vi "AB_900_1000_Project_App_Info.vi"(6 "dataForPrevious in":T1, 7 "action":T2, 8 "error in (no error)":errorcluster, 10 "applicationInfo in":T3, 11 "Object In":T4) -> (0 "error out":errorcluster, 2 "Application info":T3, 3 "Object Out":T4, 4 "dataFromPrevious":T1)   [LabVIEW 2020]
uses:
  <resource>/Framework/Providers/API/ItemRef.ctl
  <vilib>/AppBuilder/RW_Project/AB_RW_Project_PropBag_Action.ctl
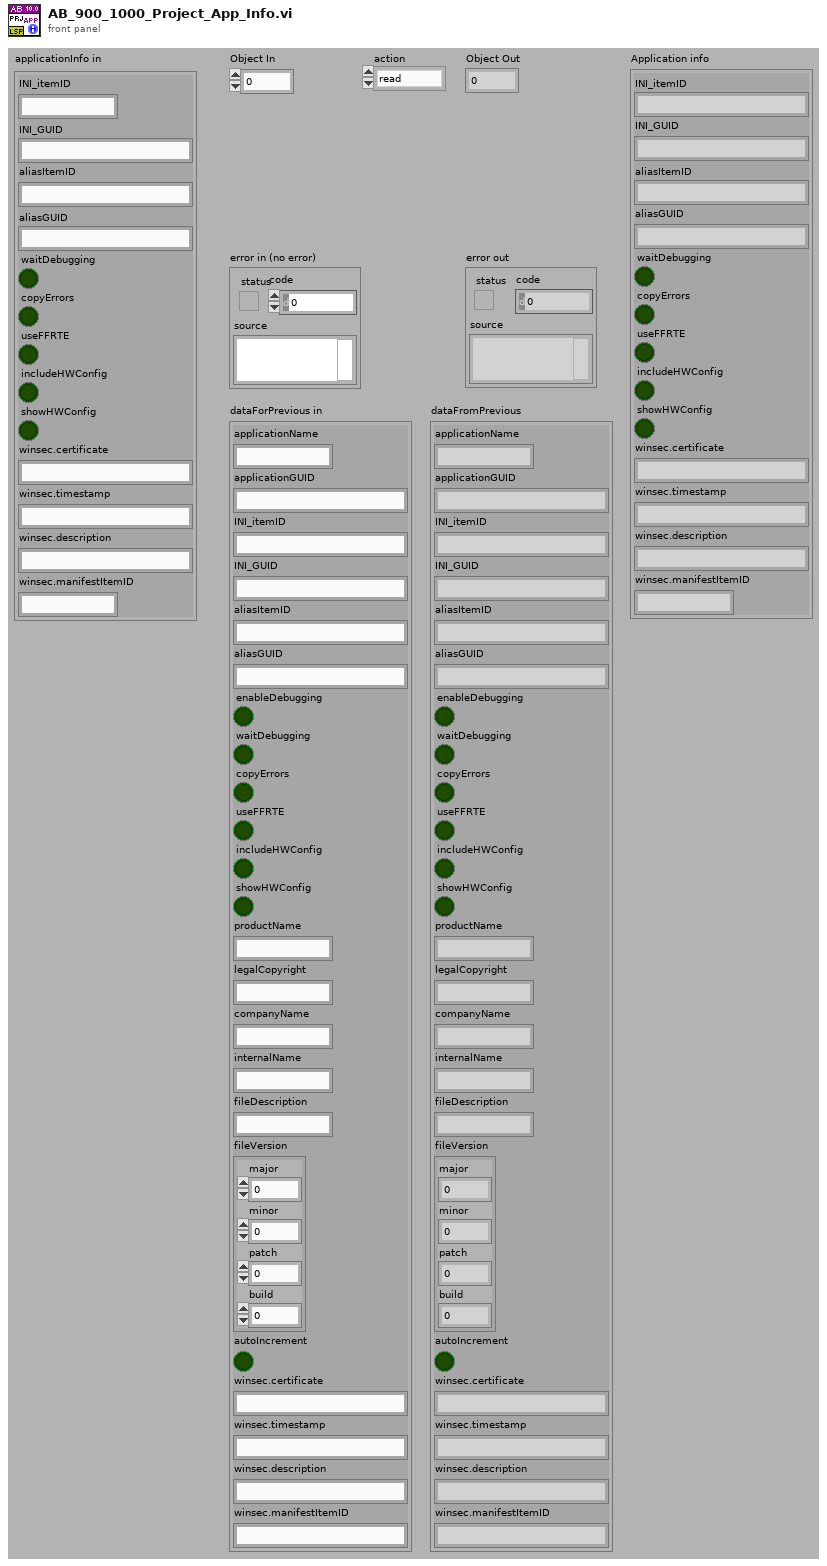
[diagram p1: front panel]
types:
  T1 = cluster{"applicationName":string, "applicationGUID":string, "INI_itemID":string, "INI_GUID":string, "aliasItemID":string, "aliasGUID":string, "enableDebugging":bool, "waitDebugging":bool, "copyErrors":bool, "useFFRTE":bool, "includeHWConfig":bool, "showHWConfig":bool, "productName":string, "legalCopyright":string, "companyName":string, "internalName":string, "fileDescription":string, "fileVersion":cluster{"major":u16, "minor":u16, "patch":u16, "build":u16}, "autoIncrement":bool, "winsec.certificate":string, "winsec.timestamp":string, "winsec.description":string, "winsec.manifestItemID":string}
  T2 = typedef "AB_RW_Project_PropBag_Action.ctl" = enum16{"read", "write", "clear", "readPrevious", "writePrevious", "clearPrevious"}
  T3 = cluster{"INI_itemID":string, "INI_GUID":string, "aliasItemID":string, "aliasGUID":string, "waitDebugging":bool, "copyErrors":bool, "useFFRTE":bool, "includeHWConfig":bool, "showHWConfig":bool, "winsec.certificate":string, "winsec.timestamp":string, "winsec.description":string, "winsec.manifestItemID":string}
  T4 = typedef "ItemRef.ctl" = u64
  T5 = cluster{"[0]":i32, "[1]":i32, "[2]":i32, "[3]":i32}
  T6 = cluster{"major":u16, "minor":u16, "patch":u16, "build":u16}
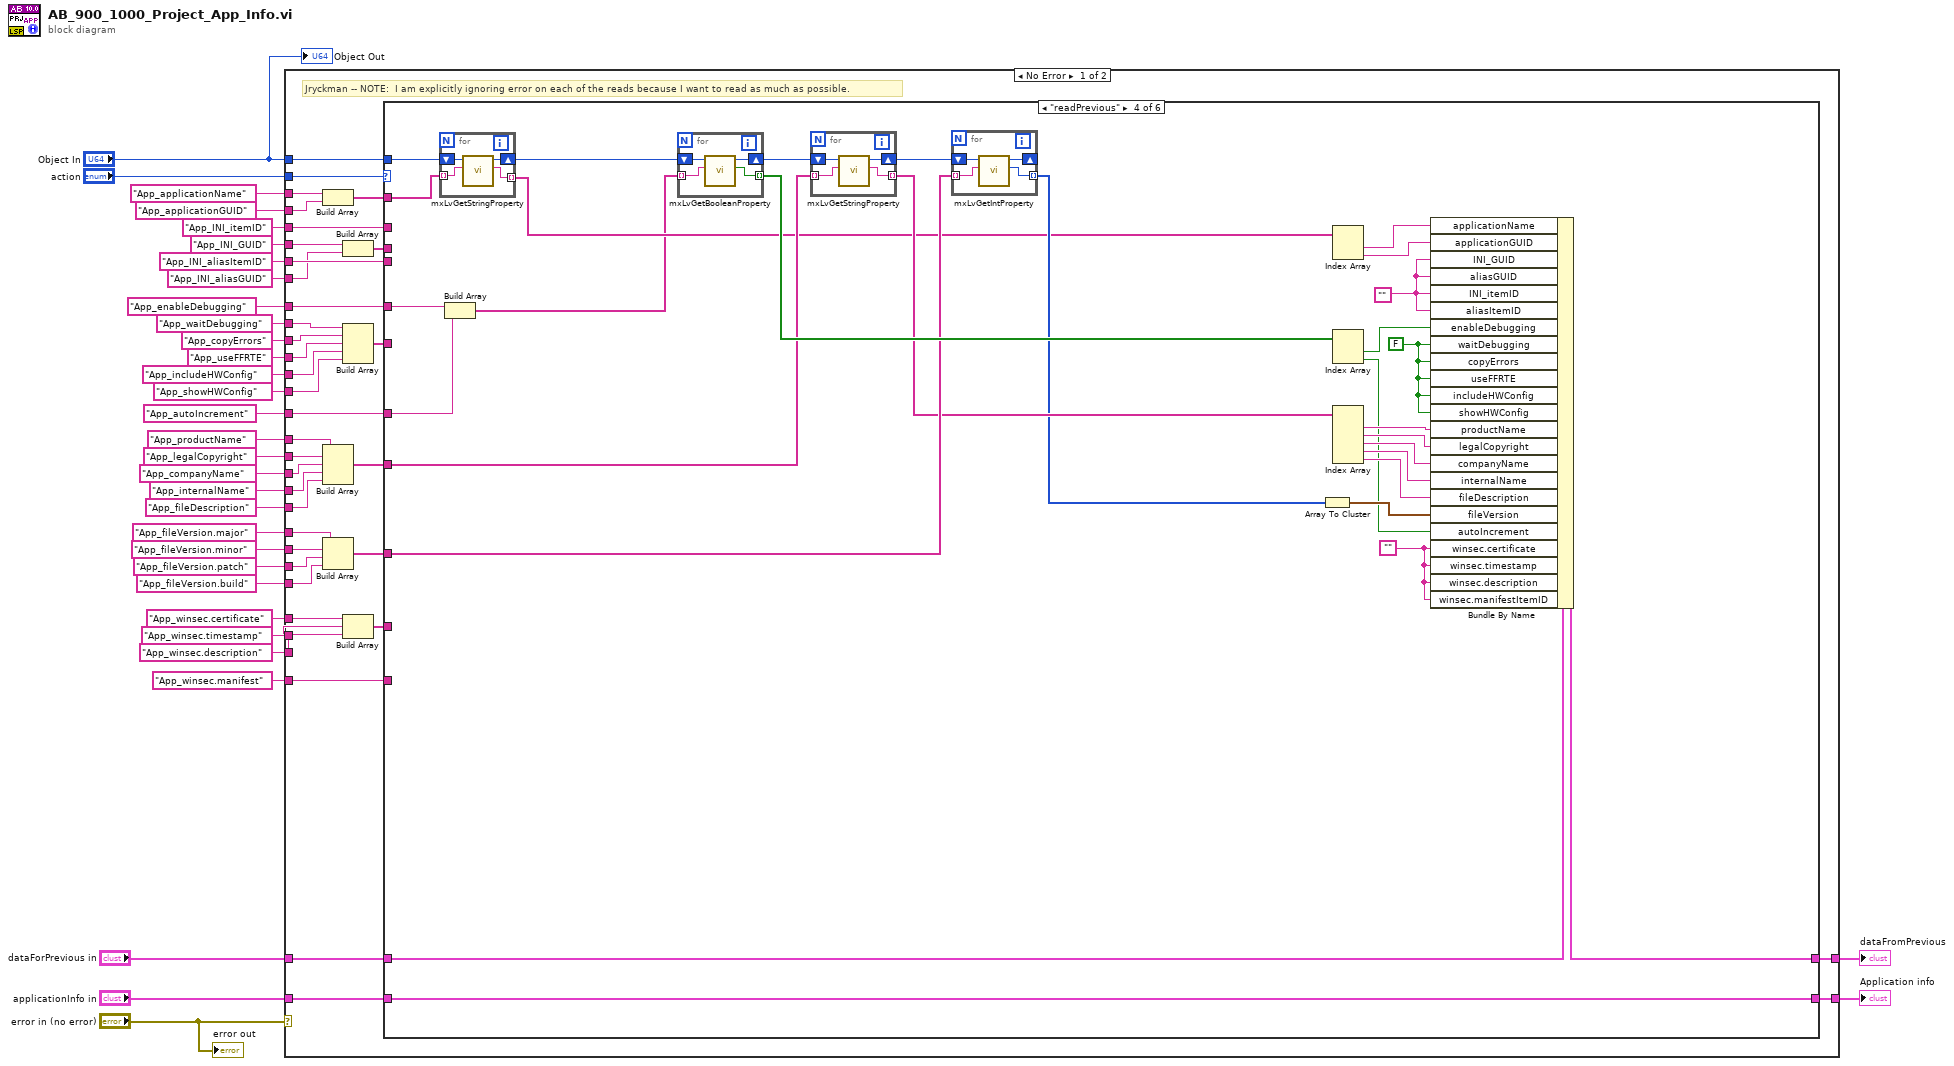
[diagram p0: block diagram]
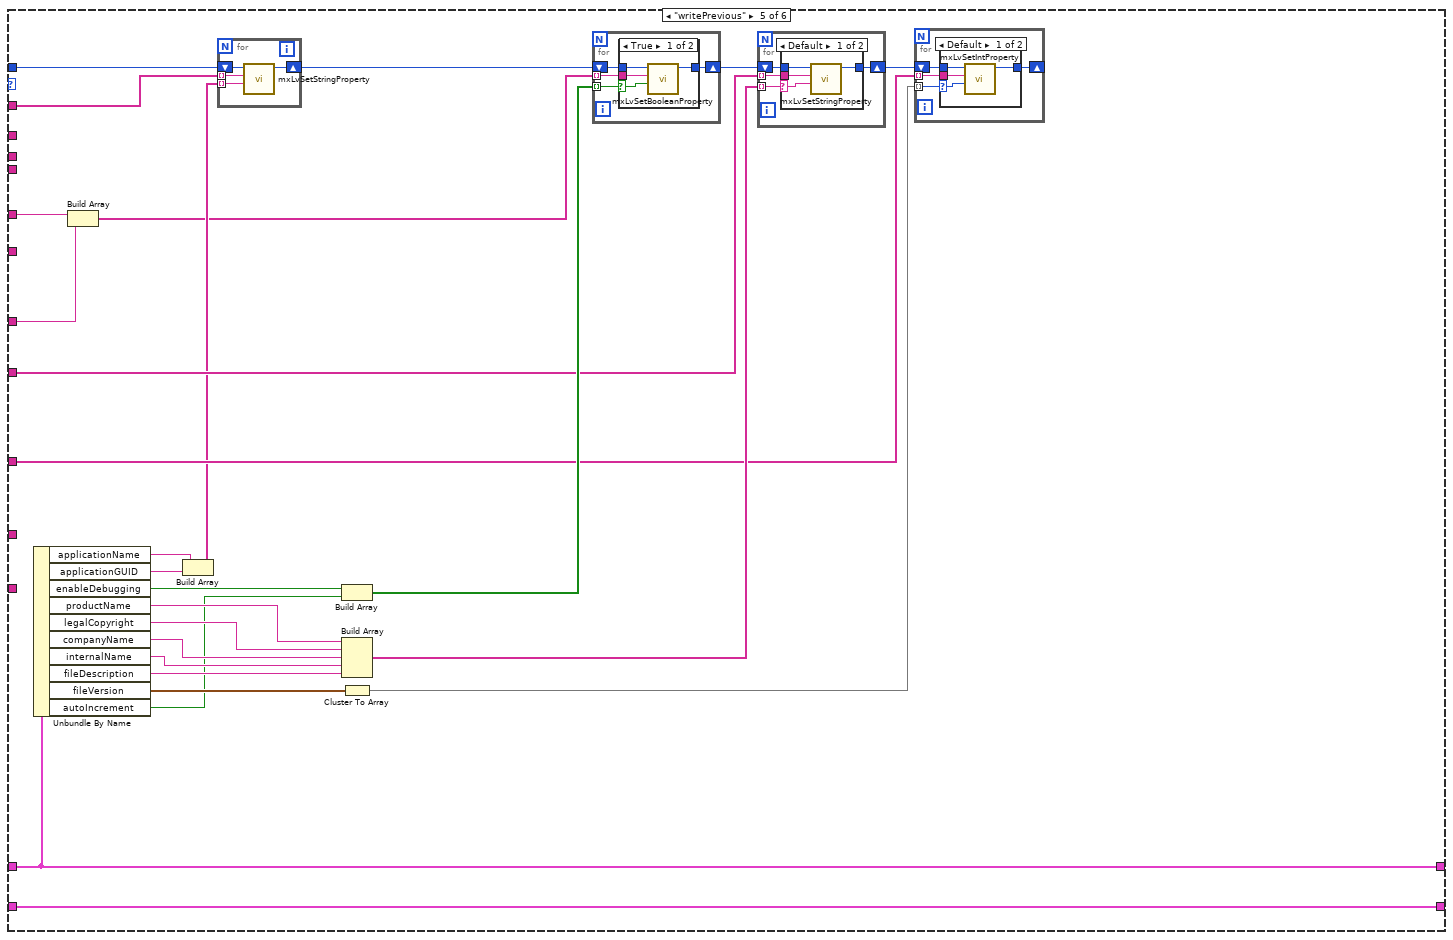
[diagram p5: hidden frame]
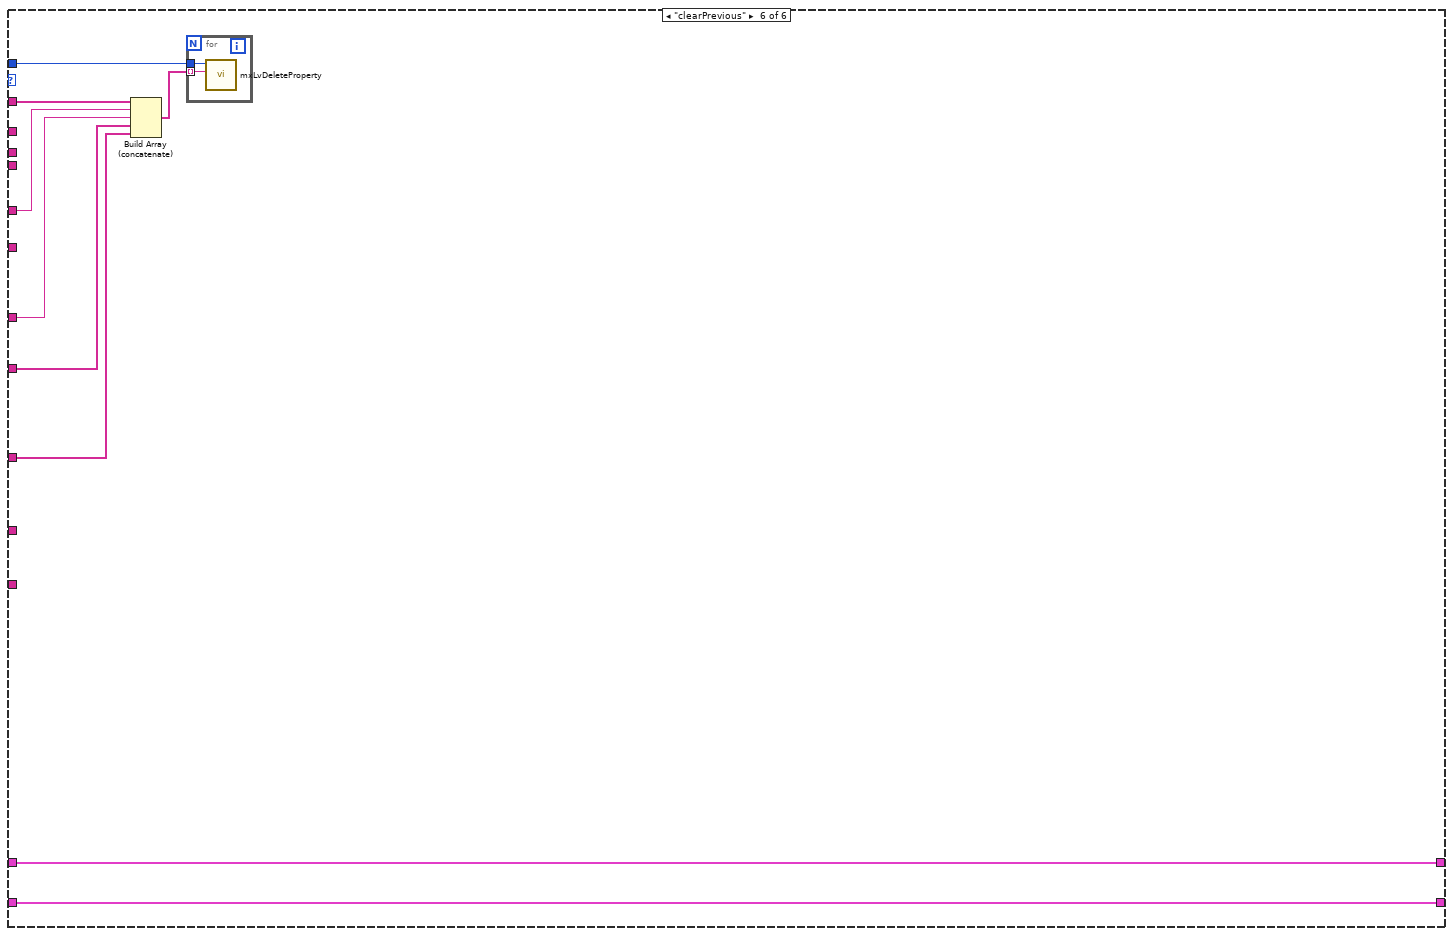
[diagram p9: hidden frame]
diagram:
  n1 = case shown="No Error" "error in (no error)" {
    tunnel: "Object In" -> [w71 _]
    tunnel: [w50 _] -> w31
    tunnel: "applicationInfo in" -> [w56 _]
    tunnel: "App_applicationName" ("Tag") -> [w37 _]
    tunnel: "App_INI_itemID" ("Tag") -> [w70 _]
    tunnel: "App_INI_aliasItemID" ("Tag") -> [w69 _]
    tunnel: "App_enableDebugging" ("Tag") -> [w39 _]
    tunnel: "App_waitDebugging" ("Tag") -> [w68 _]
    tunnel: "App_copyErrors" ("Tag") -> [w67 _]
    tunnel: "App_useFFRTE" ("Tag") -> [w66 _]
    tunnel: "App_includeHWConfig" ("Tag") -> [w65 _]
    tunnel: "App_showHWConfig" ("Tag") -> [w64 _]
    tunnel: "App_productName" ("Tag") -> [w61 _]
    tunnel: "App_legalCopyright" ("Tag") -> [w62 _]
    tunnel: "App_companyName" ("Tag") -> [w60 _]
    tunnel: "App_internalName" ("Tag") -> [w59 _]
    tunnel: "App_fileDescription" ("Tag") -> [w58 _]
    tunnel: "App_fileVersion.major" ("Tag") -> [w54 _]
    tunnel: "App_fileVersion.minor" ("Tag") -> [w55 _]
    tunnel: "App_fileVersion.patch" ("Tag") -> [w53 _]
    tunnel: "App_fileVersion.build" ("Tag") -> [w52 _]
    tunnel: "App_autoIncrement" ("Tag") -> [w38 _]
    tunnel: "action" -> [w49 _]
    tunnel: "App_applicationGUID" ("Tag") -> [w36 _]
    tunnel: "App_INI_GUID" ("Tag") -> [w48 _]
    tunnel: "App_INI_aliasGUID" ("Tag") -> [w47 _]
    tunnel: "App_winsec.certificate" ("Tag") -> [w45 _]
    tunnel: "App_winsec.timestamp" ("Tag") -> [w44 _]
    tunnel: "App_winsec.description" ("Tag") -> [w43 _]
    tunnel: "App_winsec.manifest" ("Tag") -> [w41 _]
    tunnel: "dataForPrevious in" -> [w40 _]
    tunnel: [w34 _] -> w1
    frame No Error {
      # "Jryckman -- NOTE:  I am explicitly ignoring error on each of the reads because I want to read as much as possible."
      n2 = Build Array(w37, w36) -> (w35:string[])
      n3 = Build Array(w61, w62, w60, w59, w58) -> (w57:string[])
      n4 = Build Array(w54, w55, w53, w52) -> (w51:string[])
      n5 = Build Array(w48, w47) -> (w46:string[])
      n6 = Build Array(w68, w67, w66, w65, w64) -> (w63:string[])
      n7 = Build Array(w45, w44, w43) -> (w42:string[])
      n8 = case shown="\"readPrevious\"" w49 {
        tunnel: w71 -> [_ _ _ w94 w149 w188]
        tunnel: w70 -> [_ _ _ _ _ _]
        tunnel: w69 -> [_ _ _ _ _ _]
        tunnel: w63 -> [_ _ _ _ _ _]
        tunnel: w57 -> [_ _ _ w103 w145 w187]
        tunnel: w56 -> [w72 w75 w77 w80 w135 w189]
        tunnel: w51 -> [_ _ _ w105 w138 w186]
        tunnel: [w72 w75 w77 w80 w135 w189] -> w50
        tunnel: w46 -> [_ _ _ _ _ _]
        tunnel: w42 -> [_ _ _ _ _ _]
        tunnel: w41 -> [_ _ _ _ _ _]
        tunnel: w40 -> [w73 w74 w76 w79 w125 w181]
        tunnel: w39 -> [_ _ _ w86 w129 w183]
        tunnel: w38 -> [_ _ _ w85 w128 w182]
        tunnel: w35 -> [_ _ _ w89 w124 w184]
        tunnel: [w73 w74 w76 w78 w125 w181] -> w34
        frame "read" {
        }
        frame "write" {
        }
        frame "clear" {
        }
        frame "readPrevious" {
          w81 = ""
          w82 = FALSE ("waitDebugging")
          w87 = ""
          n9 = for {
            shift-right: [w110] -> w88
            shift-left: w94 -> [w111]
            tunnel: w89 -> [w108] mode=indexing
            tunnel: [w109] -> w93 mode=indexing
            n10 = call <resource>:"mxLvGetStringProperty.vi"("Tag"=w108, "Item"=w111) -> ("Value"=w109:string, "Item"=w110:T4)  [unwired: 1 in, 7 out]
          }
          n11 = Build Array(w86, w85) -> (w84:string[])
          n12 = for {
            shift-right: [w122] -> w104
            shift-left: w88 -> [w123]
            tunnel: w84 -> [w121] mode=indexing
            tunnel: [w120] -> w107 mode=indexing
            n13 = call <resource>:"mxLvGetBooleanProperty.vi"("Tag"=w121, "Item"=w123) -> ("Value"=w120:bool, "Item"=w122:T4)  [unwired: 1 in, 7 out]
          }
          n14 = for {
            shift-right: [w118] -> w91
            shift-left: w104 -> [w119]
            tunnel: w103 -> [w116] mode=indexing
            tunnel: [w117] -> w102 mode=indexing
            n15 = call <resource>:"mxLvGetStringProperty.vi"("Tag"=w116, "Item"=w119) -> ("Value"=w117:string, "Item"=w118:T4)  [unwired: 1 in, 7 out]
          }
          n16 = for {
            shift-right: [w114] -> _
            shift-left: w91 -> [w115]
            tunnel: w105 -> [w112] mode=indexing
            tunnel: [w113] -> w96 mode=indexing
            n17 = call <resource>:"mxLvGetIntProperty.vi"("Tag"=w112, "Item"=w115) -> ("Value"=w113:i32, "Item"=w114:T4)  [unwired: 1 in, 7 out]
          }
          n18 = Array To Cluster(array=w96) -> (cluster=w95:T5)
          n19 = Index Array(array=w93) -> (element #1=w90:string, element #2=w92:string)  [unwired: 2 in]
          n20 = Index Array(array=w107) -> (element #1=w106:bool, element #2=w83:bool)  [unwired: 2 in]
          n21 = Index Array(array=w102) -> (element #1=w101:string, element #2=w100:string, element #3=w99:string, element #4=w98:string, element #5=w97:string)  [unwired: 5 in]
          n22 = Bundle By Name(cluster=w79, "applicationName"=w90, "applicationGUID"=w92, "INI_GUID"=w87, "aliasGUID"=w87, "INI_itemID"=w87, "aliasItemID"=w87, "enableDebugging"=w106, "waitDebugging"=w82, "copyErrors"=w82, "useFFRTE"=w82, "includeHWConfig"=w82, "showHWConfig"=w82, "productName"=w101, "legalCopyright"=w100, "companyName"=w99, "internalName"=w98, "fileDescription"=w97, "fileVersion"=w95, "autoIncrement"=w83, "winsec.certificate"=w81, "winsec.timestamp"=w81, "winsec.description"=w81, "winsec.manifestItemID"=w81) -> (w78:T1)
        }
        frame "writePrevious" {
          n23 = Unbundle By Name(w125) -> ("applicationName"=w132:string, "applicationGUID"=w131:string, "enableDebugging"=w126:bool, "productName"=w143:string, "legalCopyright"=w144:string, "companyName"=w142:string, "internalName"=w141:string, "fileDescription"=w140:string, "fileVersion"=w137:T6, "autoIncrement"=w133:bool)
          n24 = Build Array(w129, w128) -> (w127:string[])
          n25 = Build Array(w132, w131) -> (w130:string[])
          n26 = for {
            tunnel: w124 -> [w151] mode=indexing
            tunnel: w130 -> [w150] mode=indexing
            shift-right: [w152] -> w148
            shift-left: w149 -> [w153]
            n27 = call <resource>:"mxLvSetStringProperty.vi"("Value (\"\")"=w150, "Tag"=w151, "Item"=w153) -> ("Item"=w152:T4)  [unwired: 2 in, 6 out]
          }
          n28 = Build Array(w126, w133) -> (w147:bool[])
          n29 = Build Array(w143, w144, w142, w141, w140) -> (w139:string[])
          n30 = Cluster To Array(cluster=w137) -> (array=w136:u16[])
          n31 = for {
            tunnel: w147 -> [w174] mode=indexing
            shift-right: [w173] -> w146
            shift-left: w148 -> [w175]
            tunnel: w127 -> [w172] mode=indexing
            n32 = case shown="True" w174 {
              selector: w174 -> [w178 _]
              tunnel: w175 -> [w179 w180]
              tunnel: w172 -> [w176 _]
              tunnel: [w177 w180] -> w173
              frame True {
                n33 = call <resource>:"mxLvSetBooleanProperty.vi"("Value (F)"=w178, "Tag"=w176, "Item"=w179) -> ("Item"=w177:T4)  [unwired: 2 in, 6 out]
              }
              frame False {
              }
            }
          }
          n34 = for {
            tunnel: w139 -> [w165] mode=indexing
            shift-right: [w164] -> w134
            shift-left: w146 -> [w166]
            tunnel: w145 -> [w163] mode=indexing
            n35 = case shown="Default" w165 {
              selector: w165 -> [w168 _]
              tunnel: w166 -> [w170 w171]
              tunnel: w163 -> [w167 _]
              tunnel: [w169 w171] -> w164
              frame Default {
                n36 = call <resource>:"mxLvSetStringProperty.vi"("Value (\"\")"=w168, "Tag"=w167, "Item"=w170) -> ("Item"=w169:T4)  [unwired: 2 in, 6 out]
              }
              frame "" {
              }
            }
          }
          n37 = for {
            tunnel: w136 -> [w156] mode=indexing
            shift-right: [w155] -> _
            shift-left: w134 -> [w157]
            tunnel: w138 -> [w154] mode=indexing
            n38 = case shown="Default" w156 {
              selector: w156 -> [w160 _]
              tunnel: w157 -> [w161 w162]
              tunnel: w154 -> [w159 _]
              tunnel: [w158 w162] -> w155
              frame Default {
                n39 = call <resource>:"mxLvSetIntProperty.vi"("Value (0)"=w160, "Tag"=w159, "Item"=w161) -> ("Item"=w158:T4)  [unwired: 2 in, 6 out]
              }
              frame 0 {
              }
            }
          }
        }
        frame "clearPrevious" {
          n40 = Build Array (concatenate)(w184, w183, w182, w187, w186) -> (w185:string[])
          n41 = for {
            tunnel: w188 -> [w191]
            tunnel: w185 -> [w190] mode=indexing
            n42 = call <resource>:"mxLvDeleteProperty.vi"("Tag"=w190, "Item"=w191) -> ()  [unwired: 1 in, 9 out]
          }
        }
      }
    }
    frame Error {
    }
  }
  "Application info" <- w31
  "dataFromPrevious" <- w1
  "Object Out" <- "Object In"
  "error out" <- "error in (no error)"
